vi "_Main.vi"   [LabVIEW 2017]
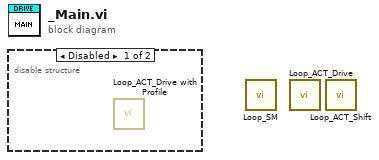
[diagram p0: block diagram]
diagram:
  n1 = disable-structure shown="Disabled" {
    frame Disabled {
      n2 = call "Loop_ACT_Drive with Profile.vi"() -> ()  [unwired: 12 in]
    }
    frame Enabled {
    }
  }
  n3 = call "Loop_SM.vi"() -> ()  [unwired: 12 in]
  n4 = call "Loop_ACT_Drive.vi"() -> ()  [unwired: 12 in]
  n5 = call "Loop_ACT_Shift.vi"() -> ()  [unwired: 12 in]
